vi "replaceTransactionTypeToken.vi"(8 "error in (no error)":errorcluster, 10 "Query In":string, 11 "Banking Transactions in":refnum<class "BankingTransactionList.lvclass">) -> (0 "error out":errorcluster, 2 "Query Out":string, 3 "Banking Transactions out":refnum<class "BankingTransactionList.lvclass">)   [LabVIEW 2018, in "BankingTransactionList.lvclass"]
uses:
  BankingTransactionList.lvclass
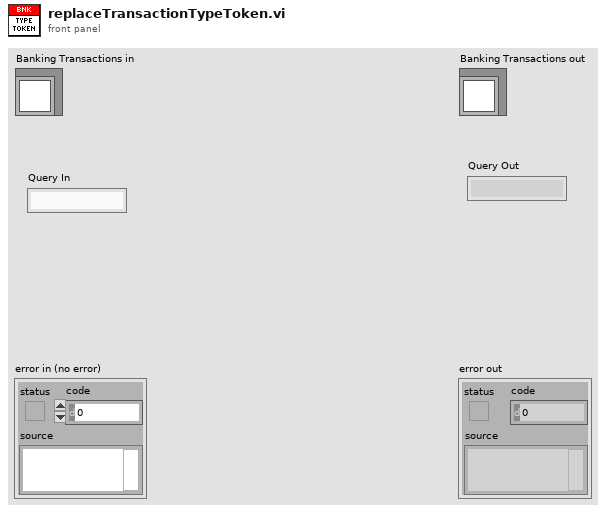
[diagram p1: front panel]
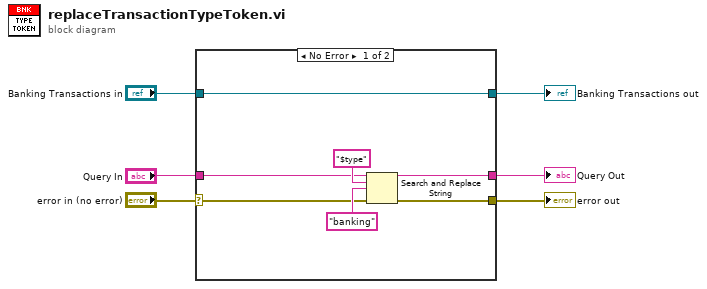
[diagram p0: block diagram]
diagram:
  n1 = case shown="No Error" "error in (no error)" {
    selector: "error in (no error)" -> [w9 w15]
    tunnel: [w8 w15] -> w5
    tunnel: [w13 w14] -> w3
    tunnel: "Banking Transactions in" -> [w13 w14]
    tunnel: "Query In" -> [w10 _]
    tunnel: [w7 _] -> w1
    frame No Error {
      n2 = Search and Replace String(input string=w10, search string="$type", replace string="banking", error in=w9) -> (result string=w7:string, error out=w8:errorcluster)  [unwired: 4 in, 2 out]
    }
    frame Error {
    }
  }
  "error out" <- w5
  "Banking Transactions out" <- w3
  "Query Out" <- w1
